vi "CountTicksBetweenSeparateLines.vi"() -> ()   [LabVIEW 2010]
uses:
  <vilib>/DAQmx/read.llb/DAQmx Read (Counter U32 1Chan 1Samp).vi
  <vilib>/DAQmx/create/channels.llb/DAQmx Create Channel (CI-Two Edge Separation).vi
  <vilib>/daqmx/miscellaneous.llb/DAQmx Fill In Error Info.vi
  C:/Program Files/National Instruments/LabVIEW 2010/resource/objmgr/daqmx.rc
panel:
  in  "D Terminal":tag="/Dev2/PFI2"
  in  "ctr C_D":tag="Dev2/ctr0" caption="Counter for C & D"
  out "ticks C_D":u32 caption="Ticks in between C & D"
  in  "C Terminal":tag="/Dev2/PFI2"
  in  "ctr B_C":tag="Dev2/ctr0" caption="Counter for B & C"
  out "ticks B_C":u32 caption="Ticks in between B & C"
  in  "Timebase Terminal":tag="/Dev2/PFI0"
  in  "B Terminal":tag="/Dev2/PFI2"
  in  "A Terminal":tag="/Dev2/PFI1"
  in  "ctr A_B":tag="Dev2/ctr0" caption="Counter for A & B"
  out "ticks A_B":u32 caption="Ticks in between A & B"
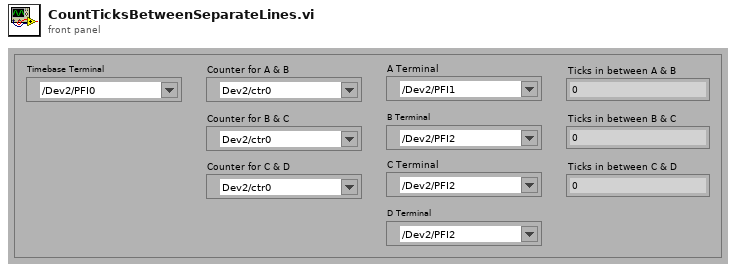
[diagram p1: front panel]
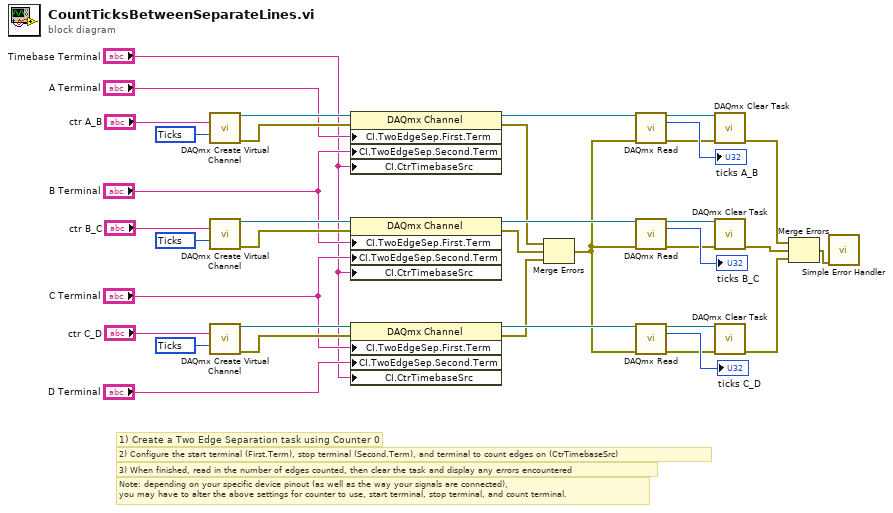
[diagram p0: block diagram]
diagram:
  w19 = 10304 items=["Seconds"=10364, "Ticks"=10304, "From Custom Scale"=10065] ("units")
  w27 = 10304 items=["Seconds"=10364, "Ticks"=10304, "From Custom Scale"=10065] ("units")
  w36 = 10304 items=["Seconds"=10364, "Ticks"=10304, "From Custom Scale"=10065] ("units")
  # "Note: depending on your specific device pinout (as well as the way your signals are connected), \nyou may have to alter the above settings for counter to use, start terminal, stop terminal, and count terminal."
  # "3) When finished, read in the number of edges counted, then clear the task and display any errors encountered"
  # "2) Configure the start terminal (First.Term), stop terminal (Second.Term), and terminal to count edges on (CtrTimebaseSrc)"
  # "1) Create a Two Edge Separation task using Counter 0"
  n1 = call-poly <vilib>:"DAQmx Create Virtual Channel.vi"("counter"="ctr A_B", "units"=w36) -> ("task out"=w35:refnum<k21>, "error out"=w34:errorcluster)  [unwired: 8 in, 4 out]
  n2 = call-poly <vilib>:"DAQmx Create Virtual Channel.vi"("counter"="ctr B_C", "units"=w27) -> ("task out"=w26:refnum<k21>, "error out"=w25:errorcluster)  [unwired: 8 in, 4 out]
  n3 = call-poly <vilib>:"DAQmx Create Virtual Channel.vi"("counter"="ctr C_D", "units"=w19) -> ("task out"=w18:refnum<k21>, "error out"=w17:errorcluster)  [unwired: 8 in, 4 out]
  n4 = property class="DAQmx Channel"(reference=w35, error in=w34, "CI.TwoEdgeSep.First.Term"="A Terminal", "CI.TwoEdgeSep.Second.Term"="B Terminal", "CI.CtrTimebaseSrc"="Timebase Terminal") -> (reference out=w32:refnum<k21>, error out=w8:errorcluster)
  n5 = property class="DAQmx Channel"(reference=w26, error in=w25, "CI.TwoEdgeSep.First.Term"="B Terminal", "CI.TwoEdgeSep.Second.Term"="C Terminal", "CI.CtrTimebaseSrc"="Timebase Terminal") -> (reference out=w24:refnum<k21>, error out=w7:errorcluster)
  n6 = property class="DAQmx Channel"(reference=w18, error in=w17, "CI.TwoEdgeSep.First.Term"="C Terminal", "CI.TwoEdgeSep.Second.Term"="D Terminal", "CI.CtrTimebaseSrc"="Timebase Terminal") -> (reference out=w15:refnum<k21>, error out=w6:errorcluster)
  n7 = Merge Errors(w8, w7, w6) -> (w5:errorcluster)
  n8 = call-poly <vilib>:"DAQmx Read.vi"("task/channels in"=w32, "error in"=w5) -> ("task out"=w30:refnum<k21>, "data"=→"ticks A_B":u32, "error out"=w29:errorcluster)  [unwired: 11 out]
  n9 = call-poly <vilib>:"DAQmx Read.vi"("task/channels in"=w24, "error in"=w5) -> ("task out"=w22:refnum<k21>, "data"=→"ticks B_C":u32, "error out"=w21:errorcluster)  [unwired: 11 out]
  n10 = call-poly <vilib>:"DAQmx Read.vi"("task/channels in"=w15, "error in"=w5) -> ("task out"=w13:refnum<k21>, "data"=→"ticks C_D":u32, "error out"=w12:errorcluster)  [unwired: 11 out]
  n11 = call <vilib>:"DAQmx Clear Task.vi"("task in"=w30, "error in"=w29) -> ("error out"=w4:errorcluster)  [unwired: 13 out]
  n12 = call <vilib>:"DAQmx Clear Task.vi"("task in"=w22, "error in"=w21) -> ("error out"=w3:errorcluster)  [unwired: 13 out]
  n13 = call <vilib>:"DAQmx Clear Task.vi"("task in"=w13, "error in"=w12) -> ("error out"=w2:errorcluster)  [unwired: 13 out]
  n14 = Merge Errors(w4, w3, w2) -> (w1:errorcluster)
  n15 = call <vilib>:"Simple Error Handler.vi"("error in (no error)"=w1) -> ()  [unwired: 1 in, 8 out]
